vi "Check If Line Exists.vi"(8 "error in (no error)":errorcluster, 10 "name to locate":string, 11 "ScaleAndLimitModule configuration in":refnum<class "ScaleAndLimitModule configuration.lvclass">) -> (0 "error out":errorcluster, 1 "index":i32, 2 "Line":T1, 3 "ScaleAndLimitModule configuration out":refnum<class "ScaleAndLimitModule configuration.lvclass">, 5 "found?":bool)   [LabVIEW 2017, in "ScaleAndLimitModule configuration.lvclass"]
uses:
  ScaleAndLimitModule configuration.lvclass
  <vilib>/NI/Tag Bus Module Framework/channel/TBM channel.lvclass
  ScaleAndLimitModule configuration.lvclass/ScaleAndLimitModule configuration.ctl
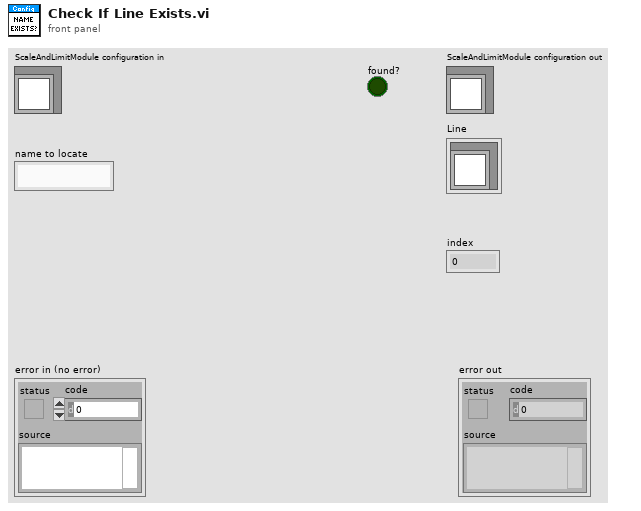
[diagram p1: front panel]
types:
  T1 = cluster{"channel":refnum<class "TBM channel.lvclass">}
  T2 = cluster{"channel":refnum<class "TBM channel.lvclass">}[]
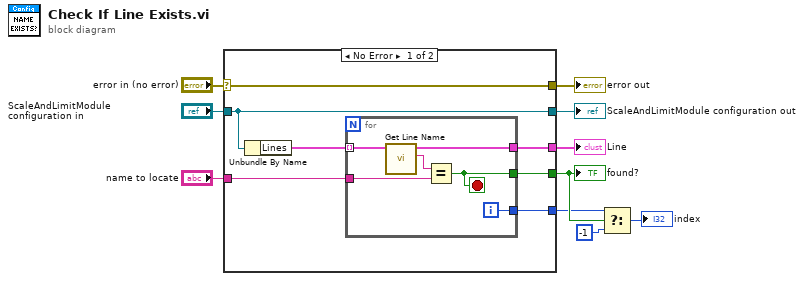
[diagram p0: block diagram]
diagram:
  n1 = case shown="No Error" "error in (no error)" {
    selector: "error in (no error)" -> [w17 w25]
    tunnel: [w17 w25] -> w9
    tunnel: [w16 w24] -> w7
    tunnel: "ScaleAndLimitModule configuration in" -> [w16 w24]
    tunnel: [w14 _] -> w6
    tunnel: "name to locate" -> [w13 _]
    tunnel: [w12 _] -> w3
    tunnel: [w11 _] -> w2
    frame No Error {
      n2 = Unbundle By Name(w16) -> ("Lines"=w15:T2)
      n3 = for {
        tunnel: w15 -> [w23] mode=indexing
        tunnel: [w22] -> w14
        tunnel: w13 -> [w20]
        tunnel: [w19] -> w12
        tunnel: [w18] -> w11
        i -> [w18]
        stop <- w19 stop-if-true
        n4 = call "Get Line Name.vi"("Line in"=w23) -> ("Name"=w21:string, "Line out"=w22:T1)  [unwired: 8 in, 1 out]
        n5 = Equal?(x=w21, y=w20) -> (x = y?=w19:bool)
      }
    }
    frame Error {
    }
  }
  "error out" <- w9
  "ScaleAndLimitModule configuration out" <- w7
  "found?" <- w3
  "Line" <- w6
  n6 = Select(t=w2, s=w3, f=-1) -> (s? t:f=→"index":i32)
